vi "globalprogram Aimé.vi"() -> ()   [LabVIEW 2019]
uses:
  <vilib>/myRIO/Common/Instrument Driver Framework/myRIO v1.0/DIO/typedefs/DIO Channels Enum.ctl
  <vilib>/myRIO/Common/Instrument Driver Framework/myRIO v1.0/DIO/typedefs/DIO Channels List.ctl
  <vilib>/myRIO/Common/Instrument Driver Framework/Utilities/typedefs/Generic FPGA Reference.ctl
  <vilib>/myRIO/Common/Instrument Driver Framework/Utilities/typedefs/myRIO v1.0 Reference.ctl
  <vilib>/myRIO/Common/Instrument Driver Framework/Utilities/typedefs/Hardware Version Enum.ctl
  <vilib>/myRIO/Common/Instrument Driver Framework/Utilities/typedefs/myRIO Generic Hardware Reference.ctl
  <vilib>/myRIO/Instrument Drivers/Onboard IO/DIO/typedefs/DIO Reference.ctl
  <vilib>/myRIO/Instrument Drivers/Onboard IO/DIO/DIO.lvlib
  <vilib>/myRIO/Instrument Drivers/Onboard IO/DIO/vis/Write.vi
  <vilib>/userDefined/High Color/nirio_resource_hc.ctl
  <vilib>/myRIO/Common/Instrument Driver Framework/myRIO v1.0/DIO/vis/myRIO v1.1 Open DIO.vi
  <vilib>/myRIO/Instrument Drivers/Onboard IO/DIO/vis/myRIO DIO Open.xnode
  <vilib>/myRIO/Common/Instrument Driver Framework/Utilities/vis/Is FPGA Ref Available.vi
  <vilib>/myRIO/Express VI/Onboard IO/DO/DO Express VI.xnode
  <vilib>/myRIO/Common/Instrument Driver Framework/Utilities/typedefs/Analog Scaling Constants.ctl
  <vilib>/myRIO/Common/Instrument Driver Framework/Utilities/typedefs/Analog Scaling Constants List.ctl
  <vilib>/myRIO/Common/Instrument Driver Framework/myRIO v1.0/AO/typedefs/AO Channels Enum.ctl
  <vilib>/myRIO/Common/Instrument Driver Framework/myRIO v1.0/AO/typedefs/AO Channels List.ctl
  <vilib>/myRIO/Instrument Drivers/Onboard IO/AO/typedefs/AO Reference.ctl
  <vilib>/myRIO/Instrument Drivers/Onboard IO/AO/AO.lvlib
  <vilib>/myRIO/Instrument Drivers/Onboard IO/AO/vis/Write.vi
  <vilib>/myRIO/Common/Instrument Driver Framework/myRIO v1.0/AO/vis/myRIO v1.1 Open AO.vi
  <vilib>/myRIO/Instrument Drivers/Onboard IO/AO/vis/myRIO AO Open.xnode
  <vilib>/myRIO/Express VI/Onboard IO/AO/AO Express VI.xnode
panel:
  in  "stop manuele bediening":bool
  in  "voorwaarts":bool
  in  "rechts draaien achteruit":bool
  in  "rechts draaien":bool
  in  "achterwaarts":bool
  in  "links draaien achteruit":bool
  in  "links draaien":bool
  in  "start manuele bediening":bool
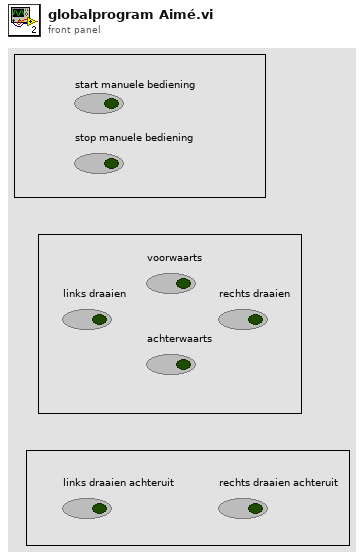
[diagram p1: front panel]
types:
  T1 = typedef "AO.lvlib/AO Reference.ctl" = cluster{"myRIO Reference":T2, "AO Channel List":T6, "AO Scaling Constant List":T8}
  T2 = typedef "myRIO Generic Hardware Reference.ctl" = cluster{"myRIO Model":T3, "myRIO Hardware Reference":T4}
  T3 = typedef "Hardware Version Enum.ctl" = enum16{"Unknown", "myRIO-1900", "myRIO-1950", "roboRIO", "NI ELVIS RIO CM", "ELVIS III"}
  T4 = typedef "myRIO v1.0 Reference.ctl" = cluster{"Generic FPGA Reference":T5, "Allow multiple opens":bool}
  T5 = typedef "Generic FPGA Reference.ctl" = refnum<k20>
  T6 = typedef "AO Channels List.ctl" = T7[]
  T7 = typedef "AO Channels Enum.ctl" = enum16{"Not Connected", "AudioOut/Left", "AudioOut/Right", "C/AO0", "C/AO1", "A/AO0", "A/AO1", "B/AO0", "B/AO1"}
  T8 = typedef "Analog Scaling Constants List.ctl" = T9[]
  T9 = typedef "Analog Scaling Constants.ctl" = cluster{"LSB Weight (Volts)":dbl, "Offset (Volts)":dbl, "Signed?":bool}
  T10 = typedef "nirio_resource_hc.ctl" = tag
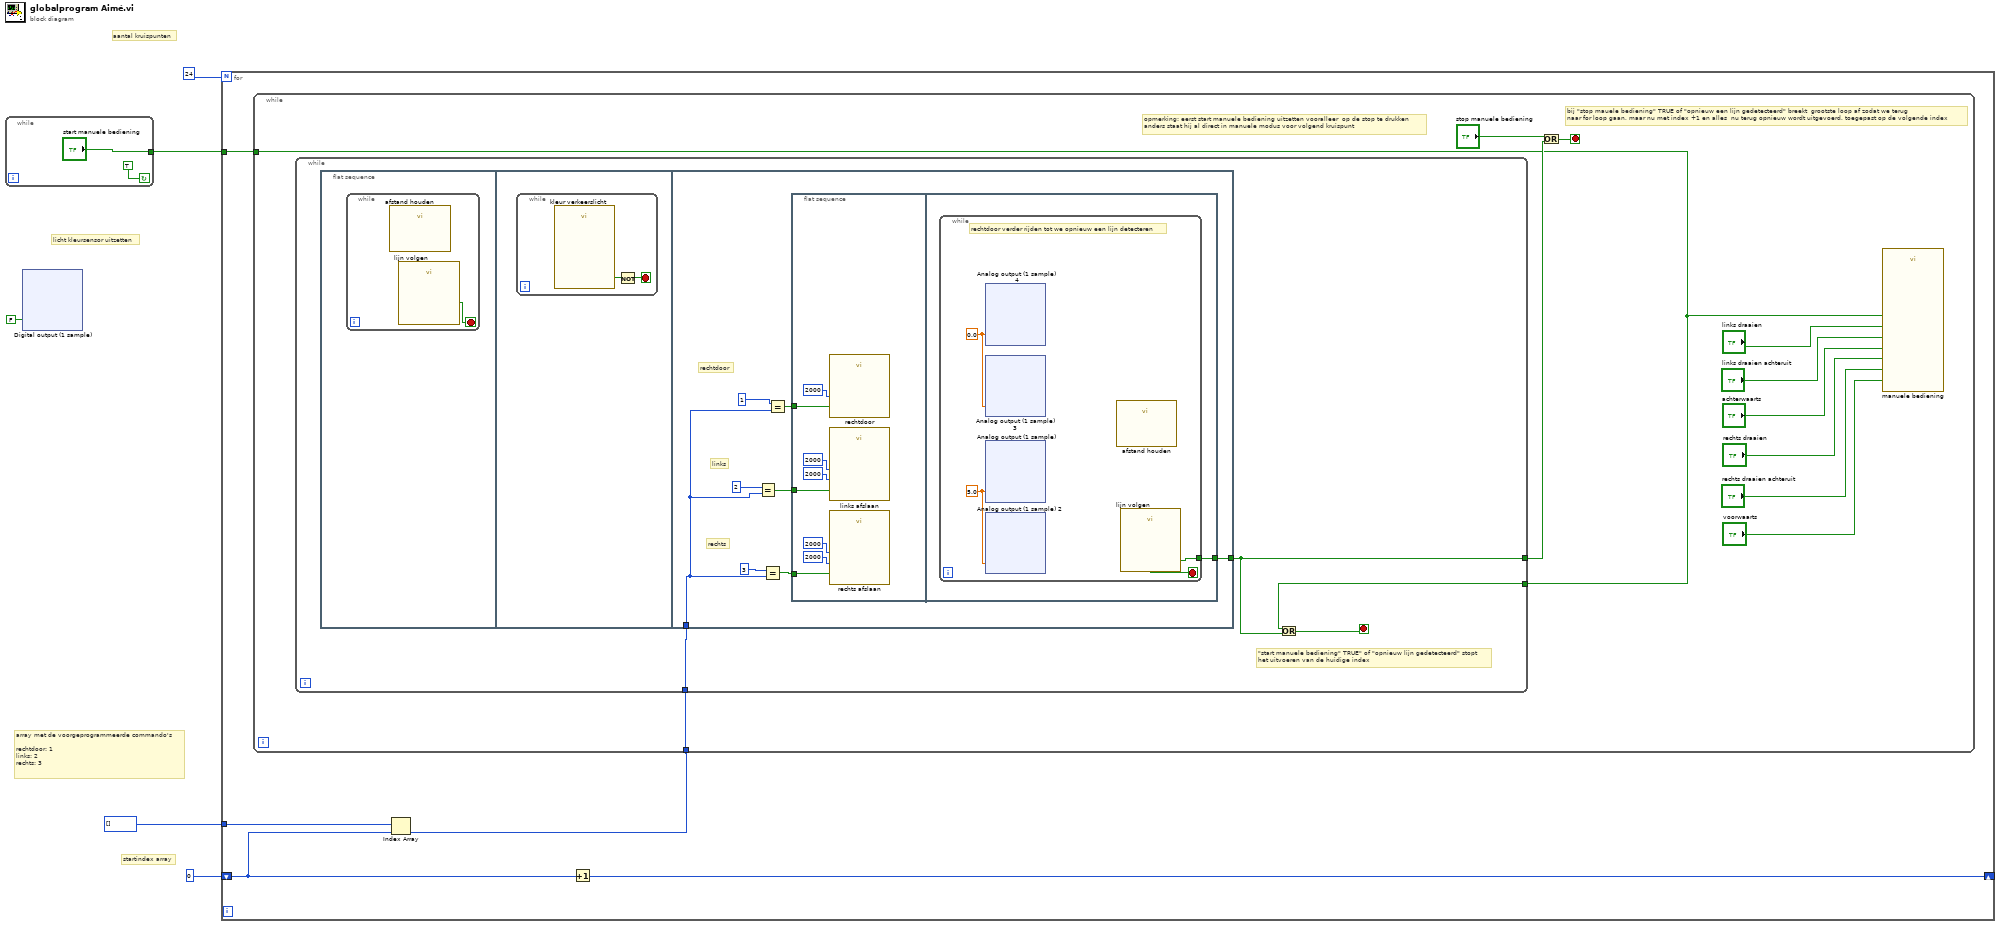
[diagram p0: block diagram]
diagram:
  # "startindex array"
  # "array met de voorgeprogrammeerde commando's\n\nrechtdoor: 1\nlinks: 2\nrechts: 3"
  # "aantal kruispunten"
  # "licht kleursensor uitzetten"
  n1 = while {
    tunnel: ["start manuele bediening"] -> w1
    stop <- TRUE continue-if-true
  }
  n2 = xnode "Digital output (1 sample)"("A/DIO2 (Pin 15)"=FALSE) -> ()  [unwired: 1 in, 1 out]
  n3 = for {
    N: 24 -> [_]
    shift-right: [w12] -> _
    shift-left: 0 -> [w11]
    tunnel: i32[] [] -> [w10]
    tunnel: w1 -> [w8]
    n4 = Index Array(array=w10, index=w11) -> (element=w9:i32)
    n5 = while {
      tunnel: w9 -> [w14]
      tunnel: w8 -> [w13]
      stop <- w17 stop-if-true
      # "opmerking: eerst start manuele bediening uitzetten vooralleer  op de stop te drukken\nanders staat hij al direct in manuele modus voor volgend kruispunt"
      # "bij \"stop mauele bediening\" TRUE of \"opnieuw een lijn gedetecteerd\" breekt  grootste loop af zodat we terug \nnaar for loop gaan, maar nu met index +1 en alles  nu terug opnieuw wordt uitgevoerd, toegepast op de volgende index"
      n6 = while {
        tunnel: [w26] -> w15
        tunnel: w14 -> [w25]
        tunnel: w13 -> [w24]
        stop <- w27 stop-if-true
        # "\"start manuele bediening\" TRUE\" of \"opnieuw lijn gedetecteerd\" stopt\nhet uitvoeren van de huidige index"
        n7 = flat-sequence {
          tunnel: w25 -> [w35]
          tunnel: [w31] -> w26
          frame #0 {
            n8 = while {
              stop <- w28 stop-if-true
              n9 = call "afstand houden.vi"() -> ()  [unwired: 12 in]
              n10 = call "lijn volgen.vi"() -> ("staat op stopstreep"=w28:bool)  [unwired: 10 in, 1 out]
            }
          }
          frame #1 {
            n11 = while {
              stop <- w29 stop-if-true
              n12 = call "kleur verkeerslicht.vi"() -> ("rood licht"=w30:bool)  [unwired: 10 in, 1 out]
              n13 = Not(x=w30) -> (.not. x?=w29:bool)
            }
          }
          frame #2 {
            # "rechts"
            # "links"
            # "rechtdoor"
            n14 = Equal?(x=2, y=w35) -> (x = y?=w33:bool)
            n15 = Equal?(x=3, y=w35) -> (x = y?=w32:bool)
            n16 = Equal?(x=1, y=w35) -> (x = y?=w38:bool)
            n17 = flat-sequence {
              tunnel: w38 -> [w46]
              tunnel: w33 -> [w44]
              tunnel: w32 -> [w45]
              tunnel: [w47] -> w31
              frame #0 {
                n18 = call "rechtdoor.vi"("Boolean"=w46, "aantal ms rijden voorbij stopstreep"=2000) -> ()  [unwired: 10 in]
                n19 = call "links afslaan.vi"("Boolean"=w44, "aantal ms rechtdoor"=2000, "aantal ms draaien"=2000) -> ()  [unwired: 9 in]
                n20 = call "rechts afslaan.vi"("Boolean"=w45, "aantal ms rechtdoor"=2000, "aantal ms draaien"=2000) -> ()  [unwired: 9 in]
              }
              frame #1 {
                n21 = while {
                  tunnel: [w48] -> w47
                  stop <- w48 stop-if-true
                  w49 = 0.0
                  w50 = 5.0
                  # "rechtdoor verder rijden tot we opnieuw een lijn detecteren"
                  n22 = xnode "Analog output (1 sample) 4"("B/AO1 (Pin 4)"=w49) -> ()  [unwired: 1 in, 1 out]
                  n23 = xnode "Analog output (1 sample) 3"("A/AO1 (Pin 4)"=w49) -> ()  [unwired: 1 in, 1 out]
                  n24 = xnode "Analog output (1 sample)"("A/AO0 (Pin 2)"=w50) -> ()  [unwired: 1 in, 1 out]
                  n25 = xnode "Analog output (1 sample) 2"("B/AO0 (Pin 2)"=w50) -> ()  [unwired: 1 in, 1 out]
                  n26 = call "afstand houden.vi"() -> ()  [unwired: 12 in]
                  n27 = call "lijn volgen.vi"() -> ("lijn gedetecteerd"=w48:bool)  [unwired: 10 in, 1 out]
                }
              }
            }
          }
        }
        n28 = Or(x=w24, y=w26) -> (x .or. y?=w27:bool)
      }
      n29 = Or(x="stop manuele bediening", y=w15) -> (x .or. y?=w17:bool)
      n30 = call "manuele bediening.vi"("voorwaarts"="voorwaarts", "achterwaarts"="achterwaarts", "rechts draaien achteruit"="rechts draaien achteruit", "links draaien"="links draaien", "rechts draaien"="rechts draaien", "manuele bediening"=w13, "links draaien achteruit"="links draaien achteruit") -> ()  [unwired: 9 in]
    }
    n31 = Increment(x=w11) -> (x+1=w12:i32)
  }
